vi "testing_idnQuery.vi"() -> ()   [LabVIEW 2015, in "Tausand AB1000.lvlib"]
uses:
  <instrlib>/Tausand AB1000/Tausand AB1000.lvlib
panel:
  out "length":i32
  out "error out":errorcluster
  in  "VISA resource name":refnum<visa-resource-name>
  out "IDN out":string
  out "timed out?":bool
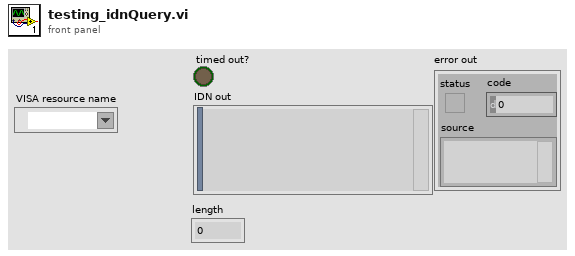
[diagram p1: front panel]
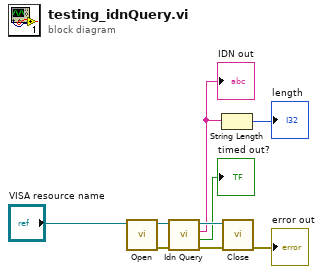
[diagram p0: block diagram]
diagram:
  n1 = call <instrlib>:"Open.vi"("VISA resource name"="VISA resource name") -> ("error out"=w9:errorcluster, "VISA resource name out"=w8:refnum<visa-resource-name>)  [unwired: 9 in]
  n2 = call <instrlib>:"Idn Query.vi"("error in (no error)"=w9, "VISA Refnum in"=w8) -> ("error out"=w6:errorcluster, "timed out?"=→"timed out?":bool, "IDN out"=w2:string, "VISA Refnum out"=w7:refnum<visa-resource-name>)  [unwired: 6 in]
  "IDN out" <- w2
  n3 = String Length(string=w2) -> (length=→"length":i32)
  n4 = call <instrlib>:"Close.vi"("error in (no error)"=w6, "VISA resource name"=w7) -> ("error out"=→"error out":errorcluster)  [unwired: 9 in]
